vi "filters_save_xml.vi"(8 "error in":errorcluster, 10 "base path":path, 11 "Filter Cluster":T1) -> (0 "error out":errorcluster)   [LabVIEW 2012]
uses:
  filters.ctl
  <vilib>/Utility/xml.llb/Write to XML File(string).vi
panel:
  # "Regions of Interest -->"
  # "Shots\n   |\n  V"
  # "Regions of Interest -->"
  # "Shots\n   |\n  V"
  # "Counters -->"
  # "Counter\n    bins\n       |\n      V"
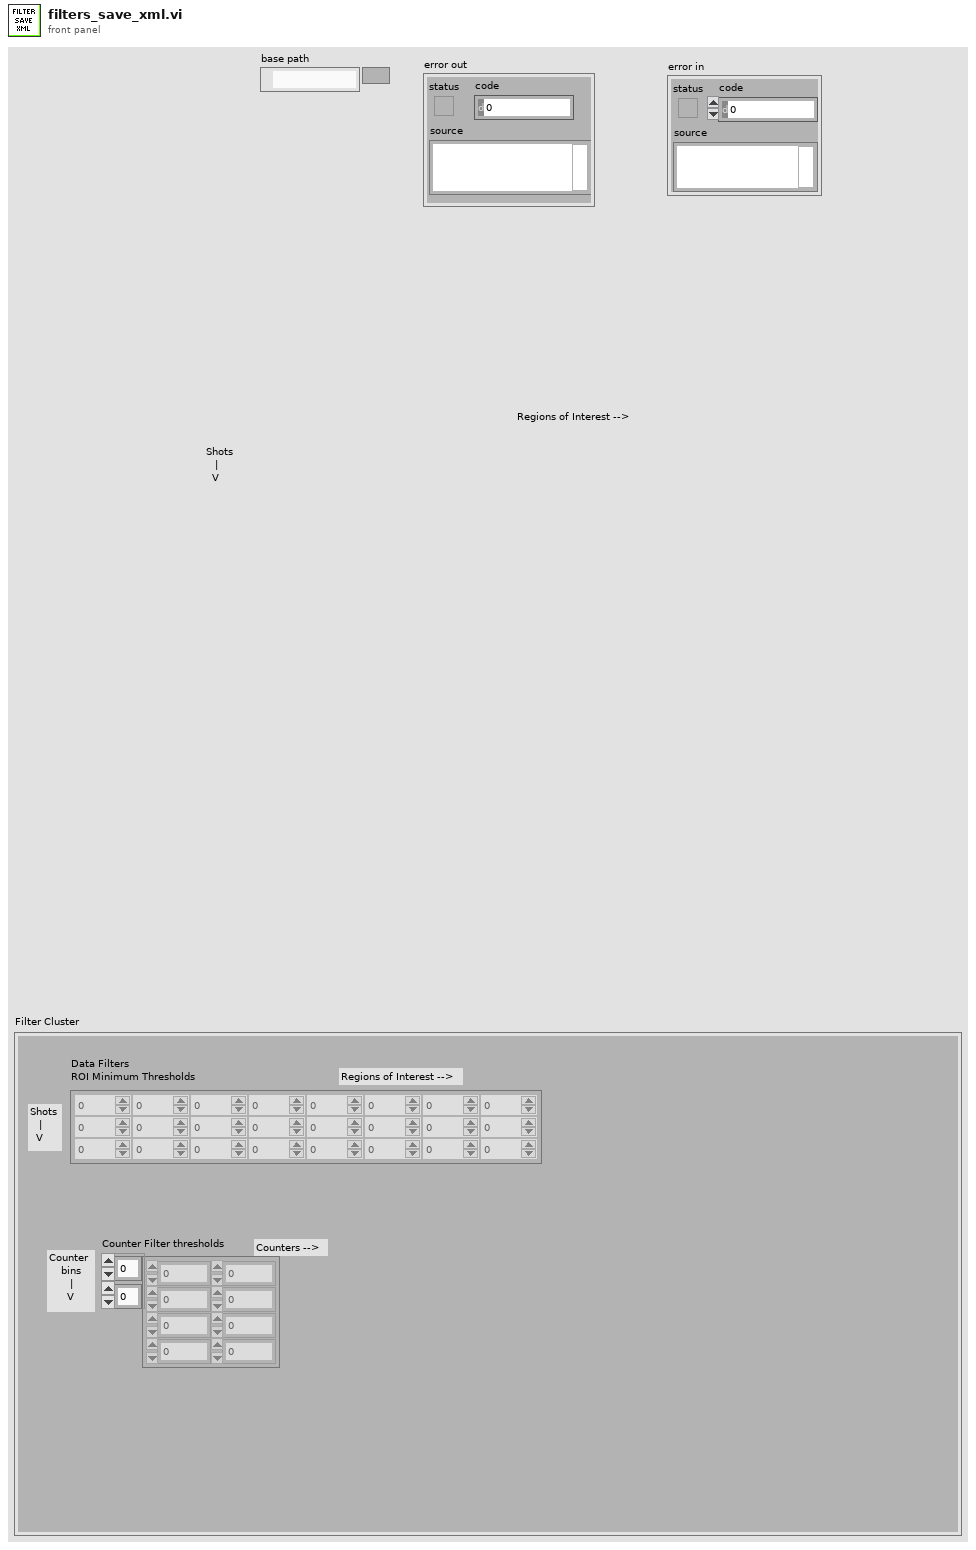
[diagram p1: front panel]
types:
  T1 = typedef "filters.ctl" = cluster{"Counter Filter thresholds":u32[][], "Data Filters\nROI Minimum Thresholds":u64[][]}
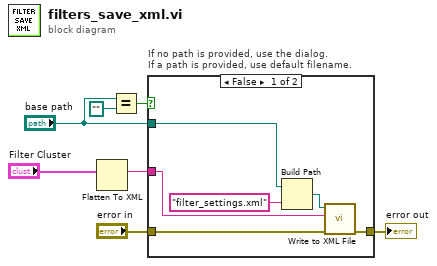
[diagram p0: block diagram]
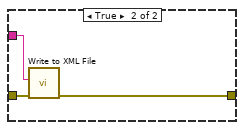
[diagram p2: hidden frame]
diagram:
  n1 = Flatten To XML(anything="Filter Cluster") -> (xml string=w2:string)
  n2 = Equal?(x="base path", y=path "") -> (x = y?=w5:bool)
  n3 = case "If no path is provided, use the dialog.\nIf a path is provided, use default filename." shown="False" w5 {
    tunnel: [w9 w15] -> w6
    tunnel: "base path" -> [w12 _]
    tunnel: "error in" -> [w10 w16]
    tunnel: w2 -> [w8 w14]
    frame False {
      n4 = Build Path(base path=w12, name or relative path="filter_settings.xml") -> (appended path=w11:path)
      n5 = call-poly <vilib>:"Write to XML File.vi"("error in (no error)"=w10, "XML Input"=w8, "XML File Path"=w11) -> ("error out"=w9:errorcluster)  [unwired: 6 in, 2 out]
    }
    frame True {
      n6 = call-poly <vilib>:"Write to XML File.vi"("error in (no error)"=w16, "XML Input"=w14) -> ("error out"=w15:errorcluster)  [unwired: 7 in, 2 out]
    }
  }
  "error out" <- w6
